vi "Pulse CS Line Script.vi"(8 "error in (no error)":errorcluster, 9 "CS line number (0)":u8, 10 "pulse width delay [ms] (0)":u8, 11 "spi script reference in":T1) -> (0 "error out":errorcluster, 3 "spi script reference out":T1)   [LabVIEW 2013, in "DDS.lvlib"]
doc: "Pulses the given CS line high then low with pulse width and preceding delay time given by pulse width delay."
uses:
  <vilib>/ni845x/ni845x.llb/ni845xSpiScriptControl.ctl
  <vilib>/ni845x/ni845x.llb/NI-845x SPI Script Ms Delay.vi
  DDS.lvlib
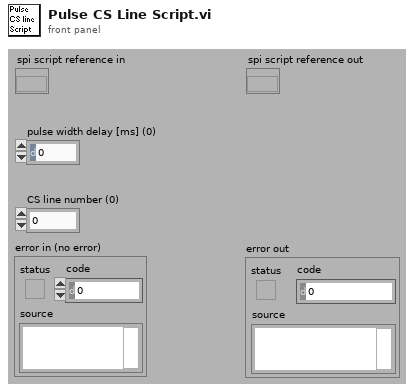
[diagram p1: front panel]
types:
  T1 = typedef "ni845xSpiScriptControl.ctl" = refnum<k20>
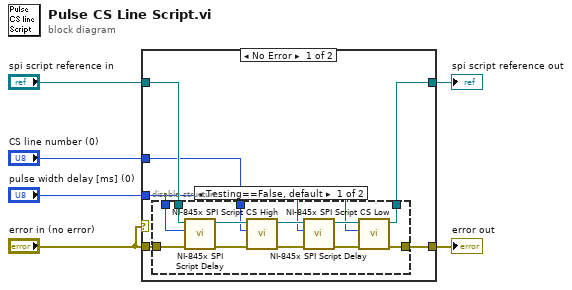
[diagram p0: block diagram]
diagram:
  n1 = case shown="No Error" "error in (no error)" {
    tunnel: [w12 w27] -> w6
    tunnel: [w11 w28] -> w5
    tunnel: "error in (no error)" -> [w10 w28]
    tunnel: "pulse width delay [ms] (0)" -> [w9 _]
    tunnel: "spi script reference in" -> [w8 w27]
    tunnel: "CS line number (0)" -> [w7 _]
    frame No Error {
      n2 = disable-structure shown="Testing==False, default" {
        disable-tunnel: [w18 w25] -> w12
        disable-tunnel: [w17 w26] -> w11
        disable-tunnel: w10 -> [w16 w26]
        disable-tunnel: w9 -> [w15 _]
        disable-tunnel: w8 -> [w14 w25]
        disable-tunnel: w7 -> [w13 _]
        frame condition #0 (active) {
          n3 = call-poly <vilib>:"NI-845x SPI Script Delay.vi"("error in (no error)"=w16, "delay in milliseconds (0)"=w15, "spi script reference in"=w14) -> ("error out"=w19:errorcluster, "spi script reference out"=w20:T1)  [unwired: 7 in]
          n4 = call <vilib>:"NI-845x SPI Script CS High.vi"("error in (no error)"=w19, "chip select (0)"=w13, "spi script reference in"=w20) -> ("error out"=w22:errorcluster, "spi script reference out"=w21:T1)  [unwired: 7 in]
          n5 = call-poly <vilib>:"NI-845x SPI Script Delay.vi"("error in (no error)"=w22, "delay in milliseconds (0)"=w15, "spi script reference in"=w21) -> ("error out"=w24:errorcluster, "spi script reference out"=w23:T1)  [unwired: 7 in]
          n6 = call <vilib>:"NI-845x SPI Script CS Low.vi"("error in (no error)"=w24, "chip select (0)"=w13, "spi script reference in"=w23) -> ("error out"=w17:errorcluster, "spi script reference out"=w18:T1)  [unwired: 7 in]
        }
        frame condition #1 {
        }
      }
    }
    frame Error {
    }
  }
  "spi script reference out" <- w6
  "error out" <- w5
